vi "Burst String to Lines.vi"(6 "preserve leading spaces":bool, 11 "read buffer":string) -> (3 "lines":string[](array[string]))   [LabVIEW 2020, in "GOLPI library.lvlib"]
uses:
  GOLPI library.lvlib
  <vilib>/Utility/error.llb/whitespace.ctl
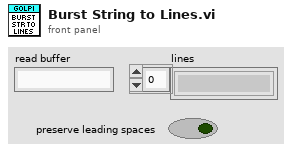
[diagram p1: front panel]
types:
  T1 = typedef "whitespace.ctl" = u16
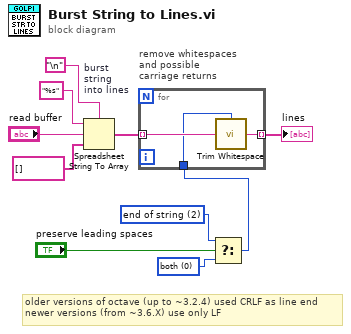
[diagram p0: block diagram]
diagram:
  w3 = T1 0 items=["both", "start of string", "end of string"] ("location (both)")
  w2 = T1 2 items=["both", "start of string", "end of string"] ("location (both)")
  # "older versions of octave (up to ~3.2.4) used CRLF as line end\nnewer versions (from ~3.6.X) use only LF"
  n1 = Spreadsheet String To Array "burst\nstring\ninto lines"(delimiter (Tab)="\n", format string="%s", spreadsheet string="read buffer", array type (2D Dbl)=string[] []) -> (array=w6:string[])
  n2 = Select(t=w2, s="preserve leading spaces", f=w3) -> (s? t:f=w1:T1)
  n3 = for "remove whitespaces\nand possible\ncarriage returns" {
    tunnel: w6 -> [w13] mode=indexing
    tunnel: [w12] -> w5 mode=indexing
    tunnel: w1 -> [w11]
    n4 = call <vilib>:"Trim Whitespace.vi"("string"=w13, "location (both)"=w11) -> ("trimmed string"=w12:string)
  }
  "lines" <- w5
